vi "startWMPStream.vi"(8 "error in (no error)":errorcluster, 11 "SoundAO in":refnum<class "SoundAO.lvclass">) -> (0 "error out":errorcluster, 3 "SoundAO out":refnum<class "SoundAO.lvclass">)   [LabVIEW 2011, in "Hardware.lvlib" / "Channels.lvlib" / "SoundAO.lvclass"]
uses:
  SoundAO.lvclass
  SoundAO.lvclass/SoundAO.ctl
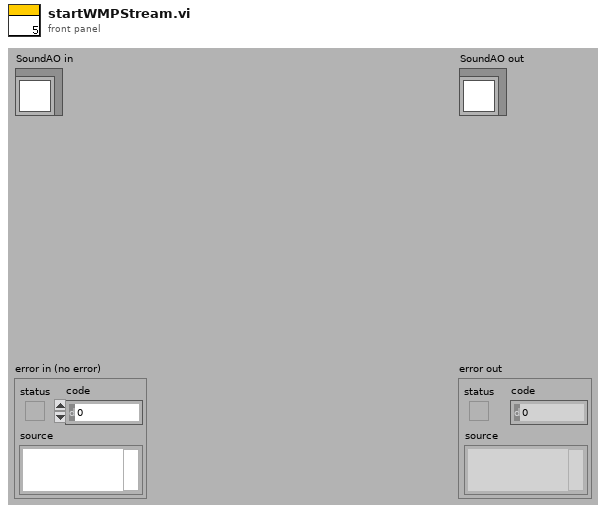
[diagram p1: front panel]
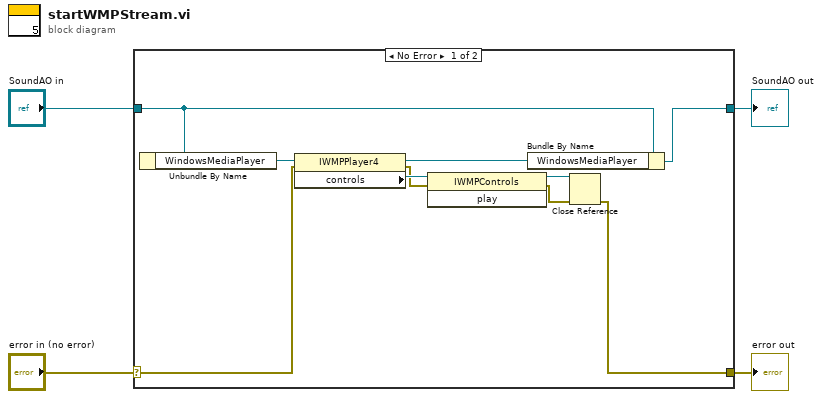
[diagram p0: block diagram]
diagram:
  n1 = case shown="No Error" "error in (no error)" {
    selector: "error in (no error)" -> [w5 w16]
    tunnel: [w6 w16] -> w3
    tunnel: [w7 w15] -> w1
    tunnel: "SoundAO in" -> [w8 w15]
    frame No Error {
      n2 = Unbundle By Name(w8) -> ("WindowsMediaPlayer"=w14:refnum<k7>)
      n3 = property class="IWMPPlayer4"(reference=w14, error in=w5) -> (reference out=w9:refnum<k7>, error out=w12:errorcluster, "controls"=w13:refnum<k7>)
      n4 = invoke class="IWMPControls" method="play"(reference=w13, error in=w12) -> (reference out=w11:refnum<k7>, error out=w10:errorcluster)  [unwired: 1 in, 1 out]
      n5 = Bundle By Name(cluster=w8, "WindowsMediaPlayer"=w9) -> (w7:refnum<class "SoundAO.lvclass">)
      n6 = Close Reference(reference=w11, error in (no error)=w10) -> (error out=w6:errorcluster)
    }
    frame Error {
    }
  }
  "error out" <- w3
  "SoundAO out" <- w1
